vi "SVPO Limit Testing (1 Ch) (SGL Waveform) with IC.vi"(7 "reset? (F)":bool, 8 "initial conditions":T2 {"timestamps"."reset" format="%<%.6X\n%x>T"; "timestamps"."first failure" format="%<%.6X\n%x>T"; "timestamps"."last failure" format="%<%.6X\n%x>T"}, 9 "lower limit":sgl=-inf format="%.2f", 10 "upper limit":sgl=inf format="%.2f", 11 "signal in":waveform(sgl)) -> (0 "final conditions":T2 {"timestamps"."reset" format="%<%.6X\n%x>T"; "timestamps"."first failure" format="%<%.6X\n%x>T"; "timestamps"."last failure" format="%<%.6X\n%x>T"}, 1 "lower limit clearance":sgl, 2 "upper limit clearance":sgl, 3 "test passed?":bool, 5 "timestamps":T1)   [LabVIEW 2017, in "SoundVib_LimitTest.lvlib"]
doc: "Performs limit testing on single-precision waveforms, single-precision scaled arrays, or double-precision scalar measurements. You can specify an upper and lower boundary of the envelope to define a pass range. This VI uses the defined pass range to test the input signal. VI outputs apply to all the tests since the last VI reset. Use this VI on embedded targets that have limited computational resources. Wire data to the <B>value in</B> input to determine the polymorphic instance to use or manually select the instance."
uses:
  <vilib>/addons/Sound and Vibration/svt_Limit Test/SoundVib_LimitTest.lvlib
  <vilib>/addons/_NISVFA/_Shared subVIs/Controls/svc_Waveform Limit State.ctl
  <vilib>/addons/_NISVFA/_Shared subVIs/Controls/svc_SGL Limit State.ctl
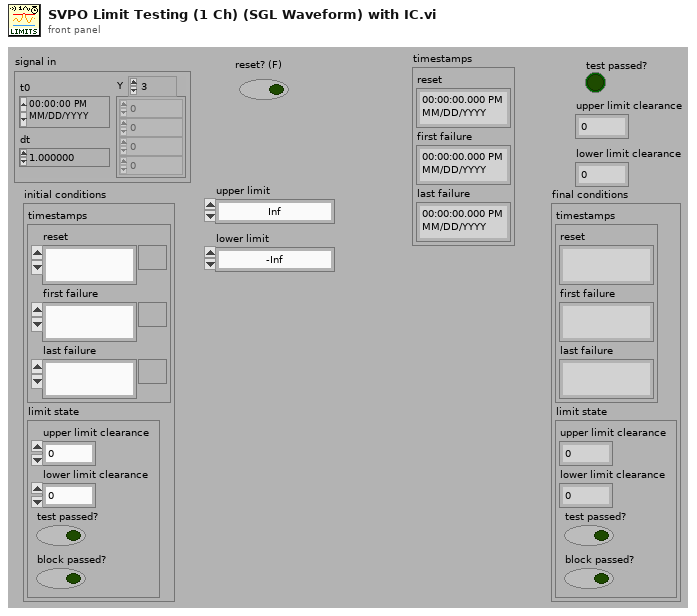
[diagram p1: front panel]
types:
  T1 = cluster{"reset":timestamp, "first failure":timestamp, "last failure":timestamp}
  T2 = typedef "svc_Waveform Limit State.ctl" = cluster{"timestamps":cluster{"reset":timestamp, "first failure":timestamp, "last failure":timestamp}, "limit state":T3}
  T3 = typedef "svc_SGL Limit State.ctl" = cluster{"upper limit clearance":sgl, "lower limit clearance":sgl, "test passed?":bool, "block passed?":bool}
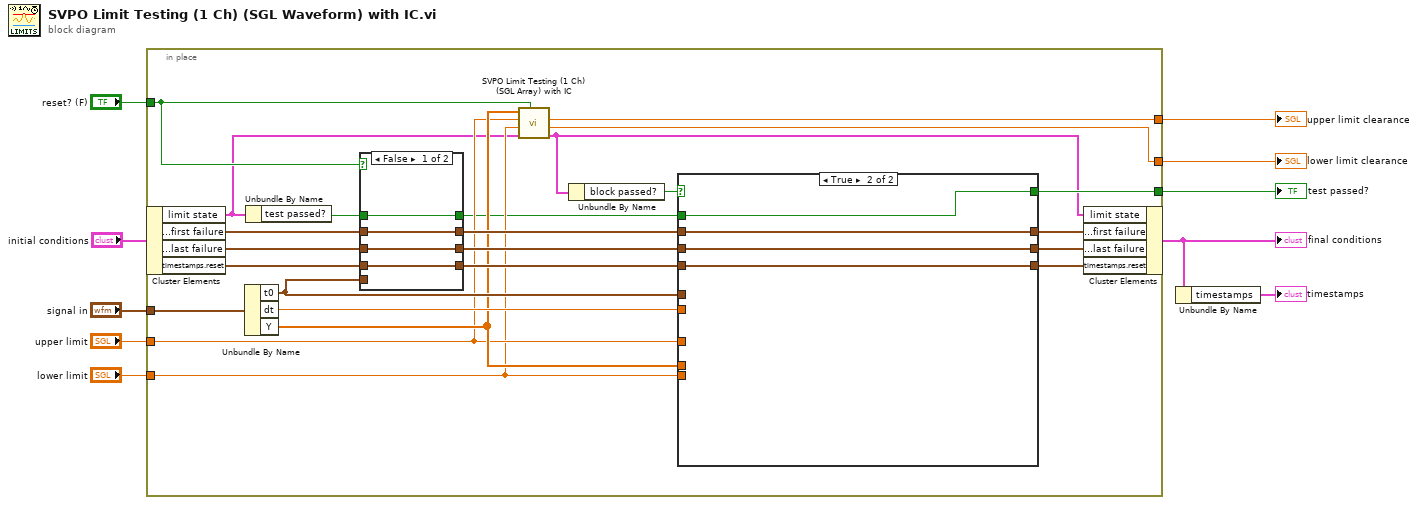
[diagram p0: block diagram]
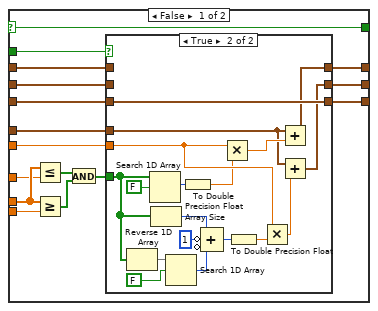
[diagram p2: hidden frame]
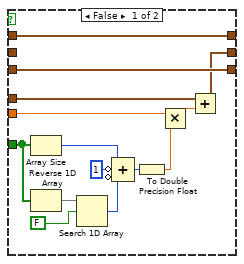
[diagram p3: hidden frame]
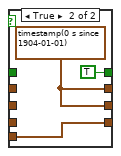
[diagram p4: hidden frame]
diagram:
  n1 = in-place {
    in-place-border: "signal in" -> [w34]
    in-place-border: "upper limit" -> [w19]
    in-place-border: "lower limit" -> [w18]
    in-place-border: "reset? (F)" -> [w20]
    in-place-border: [w17] -> w3
    in-place-border: [w16] -> w2
    in-place-border: [w22] -> w1
    n2 = in-place-cluster #1("initial conditions") -> ("limit state"=w13:T3, "timestamps.first failure"=w28:timestamp, "timestamps.last failure"=w27:timestamp, "timestamps.reset"=w26:timestamp)
    n3 = Unbundle By Name(w34) -> ("t0"=w32:timestamp, "dt"=w31:dbl, "Y"=w21:sgl[])
    n4 = Unbundle By Name(w13) -> ("test passed?"=w11:bool)
    n5 = case shown="False" w20 {
      tunnel: w26 -> [w90 _]
      tunnel: [w90 w93] -> w33
      tunnel: w32 -> [_ w93]
      tunnel: w27 -> [w88 _]
      tunnel: w28 -> [w89 _]
      tunnel: [w89 w92] -> w30
      tunnel: [w88 w92] -> w29
      tunnel: [w87 TRUE ("test passed?")] -> w12
      tunnel: w11 -> [w87 _]
      frame False {
      }
      frame True {
        w92 = timestamp(0 s since 1904-01-01) ("t0")
      }
    }
    n6 = call <vilib>:"SVPO Limit Testing (1 Ch) (SGL Array) with IC.vi"("reset? (F)"=w20, "initial conditions"=w13, "lower limit"=w18, "upper limit"=w19, "signal in"=w21) -> ("final conditions"=w15:T3, "lower limit clearance"=w16:sgl, "upper limit clearance"=w17:sgl)  [unwired: 3 in, 1 out]
    n7 = Unbundle By Name(w15) -> ("block passed?"=w14:bool)
    n8 = case shown="True" w14 {
      selector: w14 -> [w48 _]
      tunnel: w33 -> [w41 w86]
      tunnel: [w40 w86] -> w23
      tunnel: w32 -> [w50 _]
      tunnel: w31 -> [w49 _]
      tunnel: w12 -> [w35 w83]
      tunnel: [w48 w83] -> w22
      tunnel: w21 -> [w44 _]
      tunnel: w19 -> [w43 _]
      tunnel: w18 -> [w45 _]
      tunnel: [w38 w85] -> w25
      tunnel: w30 -> [w36 w85]
      tunnel: w29 -> [w39 w84]
      tunnel: [w37 w84] -> w24
      frame False {
        n9 = Less Or Equal?(x=w44, y=w43) -> (x <= y?=w47:bool[])
        n10 = Greater Or Equal?(x=w44, y=w45) -> (x >= y?=w46:bool[])
        n11 = And(x=w47, y=w46) -> (x .and. y?=w42:bool[])
        n12 = case shown="True" w35 {
          tunnel: w50 -> [w60 w75]
          tunnel: w49 -> [w59 w74]
          tunnel: w42 -> [w54 w72]
          tunnel: [w64 w80] -> w40
          tunnel: w41 -> [w64 w80]
          tunnel: w39 -> [_ _]
          tunnel: [w57 w79] -> w38
          tunnel: [w58 w76] -> w37
          tunnel: w36 -> [w57 _]
          frame False {
            n13 = Array Size(array=w54) -> (size(s)=w56:i32)
            n14 = Reverse 1D Array(array=w54) -> (reversed array=w62:bool[])
            n15 = Search 1D Array(1D array=w62, element=FALSE) -> (index of element=w53:i32)  [unwired: 1 in]
            n16 = Compound Arithmetic op=ADD(w56, invert 1 ("value"), invert w53) -> (w52:i32)
            n17 = To Double Precision Float(number=w52) -> (double precision float=w51:dbl)
            n18 = Multiply(x=w59, y=w51) -> (x*y=w61:dbl)
            n19 = Add(x=w60, y=w61) -> (x+y=w58:timestamp)
          }
          frame True {
            n20 = Reverse 1D Array(array=w72) -> (reversed array=w77:bool[])
            n21 = Search 1D Array(1D array=w72, element=FALSE) -> (index of element=w67:i32)  [unwired: 1 in]
            n22 = Array Size(array=w72) -> (size(s)=w71:i32)
            n23 = Search 1D Array(1D array=w77, element=FALSE) -> (index of element=w70:i32)  [unwired: 1 in]
            n24 = To Double Precision Float(number=w67) -> (double precision float=w68:dbl)
            n25 = Compound Arithmetic op=ADD(w71, invert 1 ("value"), invert w70) -> (w66:i32)
            n26 = Multiply(x=w74, y=w68) -> (x*y=w82:dbl)
            n27 = To Double Precision Float(number=w66) -> (double precision float=w65:dbl)
            n28 = Multiply(x=w74, y=w65) -> (x*y=w73:dbl)
            n29 = Add(x=w75, y=w82) -> (x+y=w79:timestamp)
            n30 = Add(x=w75, y=w73) -> (x+y=w76:timestamp)
          }
        }
      }
      frame True {
      }
    }
    n31 = in-place-cluster #1("limit state"=w15, "timestamps.first failure"=w25, "timestamps.last failure"=w24, "timestamps.reset"=w23) -> (w5:T2)
  }
  "final conditions" <- w5
  "upper limit clearance" <- w3
  "lower limit clearance" <- w2
  "test passed?" <- w1
  n32 = Unbundle By Name(w5) -> ("timestamps"=→"timestamps":T1)
